vi "MU Switch to BiSS Ex.vi"(8 "error in (no error)":errorcluster, 11 "handle":u64) -> (0 "error out (no error)":errorcluster, 1 "switched":bool, 2 "modea":u32, 3 "function return":u32)   [LabVIEW 2017, in "MU_3SL_interface.lvlib"]
uses:
  MU_3SL_interface.lvlib
  lib/MU_3SL_interface.dll
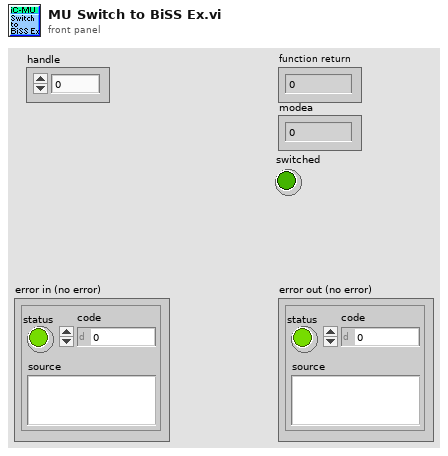
[diagram p1: front panel]
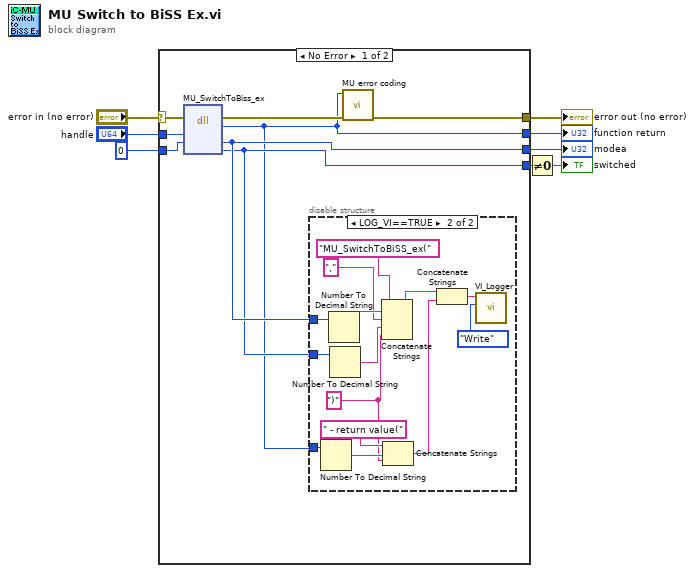
[diagram p0: block diagram]
diagram:
  n1 = case shown="No Error" "error in (no error)" {
    selector: "error in (no error)" -> [w13 w32]
    tunnel: [w9 w31] -> w8
    tunnel: "handle" -> [w16 _]
    tunnel: [w11 w31] -> w6
    tunnel: [w14 w32] -> w5
    tunnel: u32 0 ("pulMODEA") -> [w12 w31]
    tunnel: [w10 w31] -> w1
    frame No Error {
      n2 = dll-call lib="C:/Users/bes/AppData/Roaming/work/mu_9so/icsubmodules/soft_mu_3sl_master/lv_interface/lib/MU_3SL_interface**.*" fn="MU_SwitchToBiss_ex"(error in=w13, "handle"=w16, "modea"=w12) -> (error out=w15:errorcluster, "return type"=w9:u32, "modea"=w11:u32, "switched"=w10:u8)  [unwired: 4 in, 1 out]
      n3 = disable-structure shown="LOG_VI==TRUE" {
        disable-tunnel: w9 -> [_ w28]
        disable-tunnel: w11 -> [_ w23]
        disable-tunnel: w10 -> [_ w20]
        frame condition #0 {
        }
        frame condition #1 (active) {
          w17 = ")" ("string")
          n4 = Number To Decimal String(number=w28) -> (decimal integer string=w27:string)  [unwired: 1 in]
          n5 = Number To Decimal String(number=w23) -> (decimal integer string=w22:string)  [unwired: 1 in]
          n6 = Number To Decimal String(number=w20) -> (decimal integer string=w19:string)  [unwired: 1 in]
          n7 = Concatenate Strings("MU_SwitchToBiSS_ex(" ("Info in"), w22, "," ("string"), w19, w17) -> (w26:string)
          n8 = Concatenate Strings(" - return value(" ("string"), w27, w17) -> (w25:string)
          n9 = Concatenate Strings(w26, w25) -> (w24:string)
          n10 = call "VI_Logger.vi"("Action (Read)"=enum16{"Write", "Read"}."Write", "Info in"=w24) -> ()  [unwired: 8 in, 2 out]
        }
      }
      n11 = call "MU error coding.vi"("error in (no error)"=w15, "function return in"=w9) -> ("error out"=w14:errorcluster)  [unwired: 9 in]
    }
    frame Error {
    }
  }
  "function return" <- w8
  "modea" <- w6
  "error out (no error)" <- w5
  n12 = Not Equal To 0?(x=w1) -> (x != 0?=→"switched":bool)
